vi "main.vi"() -> ()   [LabVIEW 2017]
uses:
  States.ctl
  <vilib>/DAQmx/write.llb/DAQmx Write (Analog DBL 1Chan 1Samp).vi
  <vilib>/DAQmx/read.llb/DAQmx Read (Analog DBL 1Chan 1Samp).vi
  <vilib>/DAQmx/create/channels.llb/DAQmx Create Channel (AI-Voltage-Basic).vi
  <vilib>/DAQmx/create/channels.llb/DAQmx Create Channel (AO-Voltage-Basic).vi
  <vilib>/DAQmx/miscellaneous.llb/DAQmx Fill In Error Info.vi
panel:
  out "Vout2":dbl
  out "Vin":dbl
  in  "output channel":tag
  in  "input channel":tag
  in  "stop":bool
  in  "Step Voltage":dbl
  out "Vout":dbl(slide) scale=-1.0..1.0
  in  "Min Voltage":dbl
  in  "Max Voltage":dbl
  in  "Vmin (mV)":dbl
  in  "Vmax (mV)":dbl
  in  "Scan rate (mV/s)":dbl
  in  "Direction":enum16{"Cathodic", "Anodic"}(ring)
  in  "Start potential (mV)":dbl
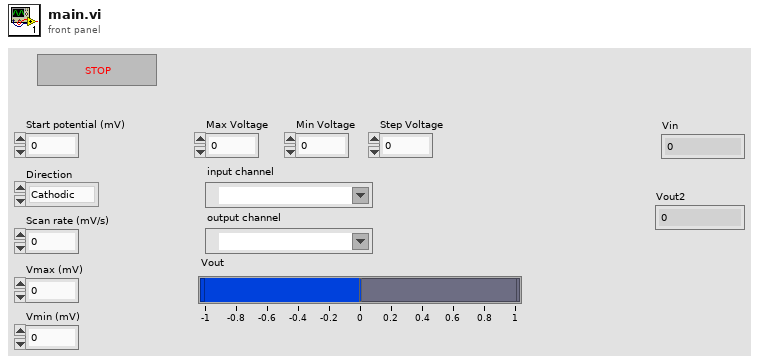
[diagram p1: front panel]
types:
  T1 = typedef "States.ctl" = enum16{"Init", "Set voltage", "Measure", "Exit"}
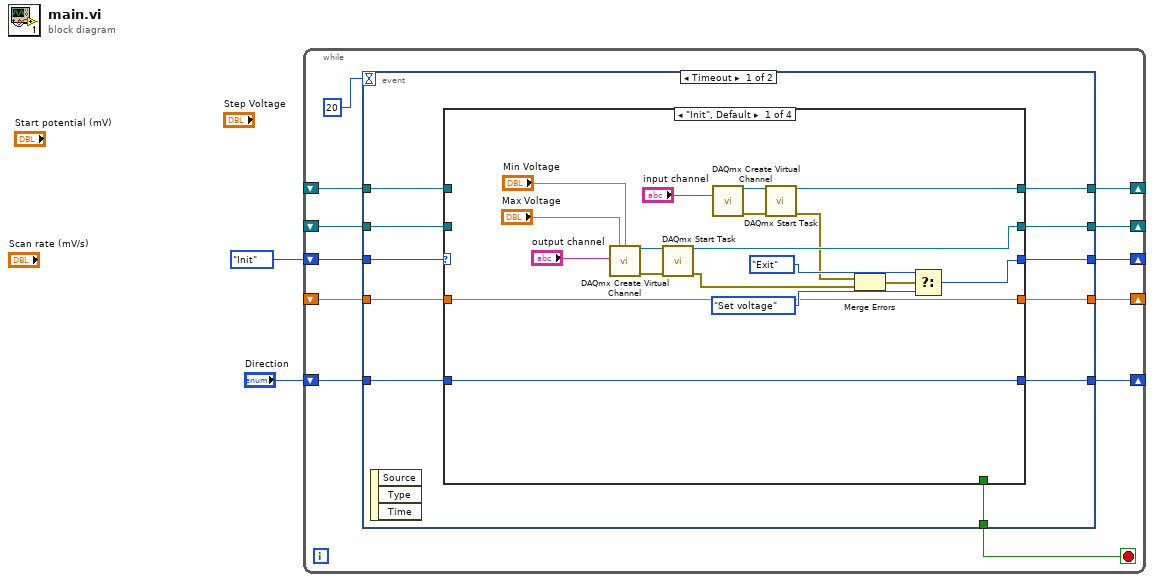
[diagram p0: block diagram]
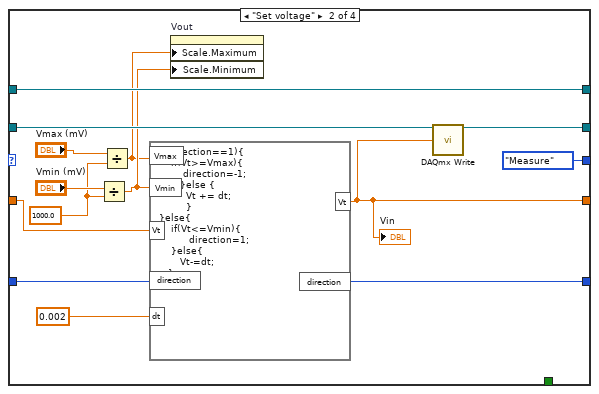
[diagram p2: hidden frame]
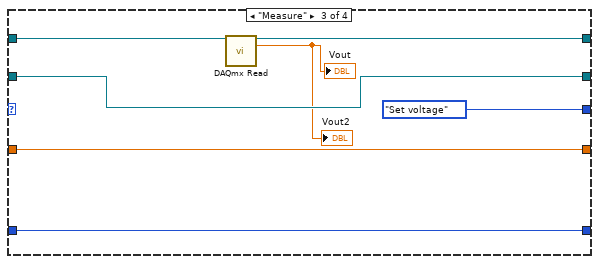
[diagram p3: hidden frame]
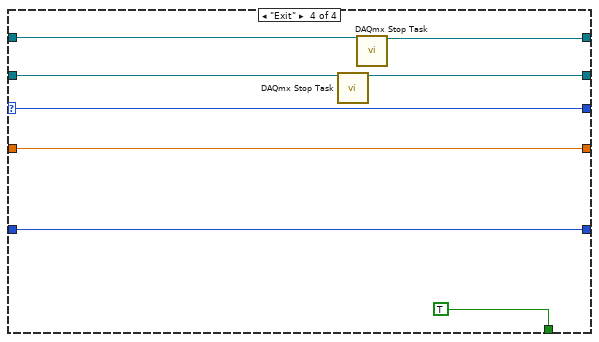
[diagram p4: hidden frame]
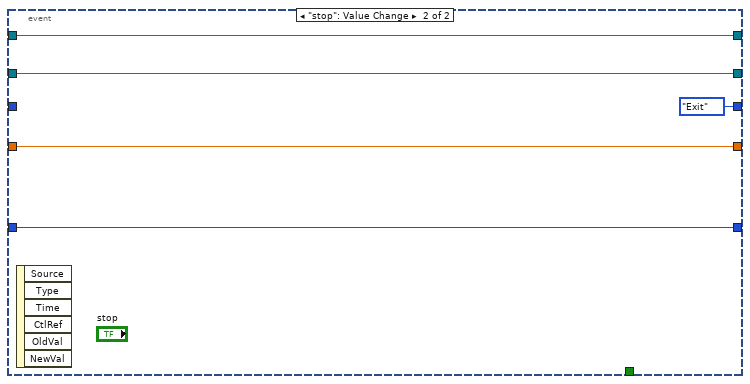
[diagram p5: hidden frame]
diagram:
  n1 = while {
    shift-right: [w12] -> _
    shift-left: _ -> [w10]
    shift-right: [w11] -> _
    shift-left: States."Init" -> [w14]
    shift-right: [w7] -> _
    shift-left: "Direction" -> [w8]
    shift-right: [w6] -> _
    shift-left: _ -> [w5]
    shift-right: [w4] -> _
    shift-left: _ -> [w3]
    stop <- w13 stop-if-true
    n2 = event shown="[0] Timeout" {
      selector: _ -> [_ _]
      dyn-events: _ -> [_ _]
      timeout: 20 -> [_ _]
      tunnel: w14 -> [w25 _]
      tunnel: [w24 _] -> w13
      tunnel: [w23 w75] -> w12
      tunnel: [w22 States."Exit"] -> w11
      tunnel: w10 -> [w21 w75]
      tunnel: w8 -> [w20 w73]
      tunnel: [w19 w73] -> w7
      tunnel: [w18 w76] -> w6
      tunnel: w5 -> [w17 w76]
      tunnel: [w16 w74] -> w4
      tunnel: w3 -> [w15 w74]
      event Timeout {
        n3 = event-data() -> ()  [unwired: 1 in, 3 out]
        n4 = case shown="\"Init\", Default" w25 {
          selector: w25 -> [_ _ _ w71]
          tunnel: [_ _ _ TRUE] -> w24
          tunnel: [w41 w55 w60 w69] -> w23
          tunnel: [w39 States."Measure" States."Set voltage" w71] -> w22
          tunnel: w21 -> [_ w56 w60 w70]
          tunnel: w20 -> [w35 w53 w63 w68]
          tunnel: [w35 w52 w63 w68] -> w19
          tunnel: [w27 w51 w61 w66] -> w18
          tunnel: w17 -> [_ w51 w62 w65]
          tunnel: [w26 w49 w58 w67] -> w16
          tunnel: w15 -> [w26 w47 w58 w67]
          frame "Init", Default {
            n5 = call-poly <vilib>:"DAQmx Create Virtual Channel.vi"("maximum value"="Max Voltage", "minimum value"="Min Voltage", "physical channels"="output channel") -> ("task out"=w43:refnum<k21>, "error out"=w42:errorcluster)  [unwired: 11 in]
            n6 = call <vilib>:"DAQmx Start Task.vi"("task/channels in"=w43, "error in"=w42) -> ("task out"=w41:refnum<k21>, "error out"=w28:errorcluster)  [unwired: 12 in]
            n7 = call-poly <vilib>:"DAQmx Create Virtual Channel.vi"("physical channels"="input channel") -> ("task out"=w32:refnum<k21>, "error out"=w31:errorcluster)  [unwired: 13 in]
            n8 = call <vilib>:"DAQmx Start Task.vi"("task/channels in"=w32, "error in"=w31) -> ("task out"=w27:refnum<k21>, "error out"=w29:errorcluster)  [unwired: 12 in]
            n9 = Merge Errors(w29, w28) -> (w30:errorcluster)
            n10 = Select(t=States."Exit", s=w30, f=States."Set voltage") -> (s? t:f=w39:T1)
          }
          frame "Set voltage" {
            w48 = 1000.0 ("y")
            n11 = Divide(x="Vmin (mV)", y=w48) -> (x/y=w45:dbl)
            n12 = Divide(x="Vmax (mV)", y=w48) -> (x/y=w44:dbl)
            n13 = formula code="if(direction==1){\n    if(Vt>=Vmax){\n        direction=-1;\n       }else { \n         Vt += dt;\n         }\n}else{\n    if(Vt<=Vmin){\n          direction=1;\n    }else{\n       Vt-=dt;      \n   }\n}"("Vmax"=w44, "Vmin"=w45, "Vt"=w47, "direction"=w53, "dt"=0.002 ("input variable")) -> ("Vt"=w49:dbl, "direction"=w52:enum16{"Cathodic", "Anodic"})
            "Vin" <- w49
            n14 = property on="Vout" class="Slide (strict)"("Scale.Maximum"=w44, "Scale.Minimum"=w45) -> ()  [unwired: 2 in, 2 out]
            n15 = call-poly <vilib>:"DAQmx Write.vi"("task/channels in"=w56, "data"=w49) -> ("task out"=w55:refnum<k21>)  [unwired: 11 in, 2 out]
          }
          frame "Measure" {
            n16 = call-poly <vilib>:"DAQmx Read.vi"("task/channels in"=w62) -> ("task out"=w61:refnum<k21>, "data"=→"Vout" →"Vout2":dbl)  [unwired: 12 in, 1 out]
          }
          frame "Exit" {
            n17 = call <vilib>:"DAQmx Stop Task.vi"("task/channels in"=w70) -> ("task out"=w69:refnum<k21>)  [unwired: 13 in, 1 out]
            n18 = call <vilib>:"DAQmx Stop Task.vi"("task/channels in"=w65) -> ("task out"=w66:refnum<k21>)  [unwired: 13 in, 1 out]
          }
        }
      }
      event "stop": Value Change {
        n19 = event-data() -> ()  [unwired: 1 in, 6 out]
      }
    }
  }
